vi "Close Device (SubVI).vi"(8 "error in (no error)":errorcluster, 11 "handle in":i64) -> (0 "error out":errorcluster, 3 "Context_handle":i64)   [LabVIEW 2015]
uses:
  libkinect_wrapper.dll
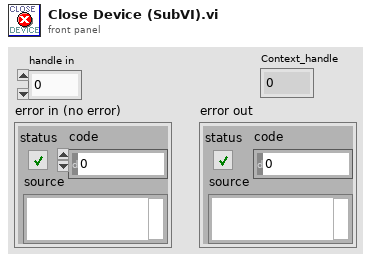
[diagram p1: front panel]
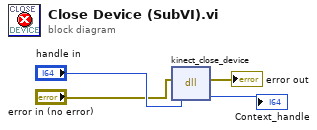
[diagram p0: block diagram]
diagram:
  n1 = dll-call lib="libkinect_wrapper.*" fn="kinect_close_device"(error in="error in (no error)", "Context_handle"="handle in") -> (error out=→"error out":errorcluster, "Context_handle"=→"Context_handle":i64)  [unwired: 3 in, 1 out]
